vi "KV_CurHead_ReadCur.vi"(10 "地址":u8=1 max=10 step=1, 11 "MyIndex":u8) -> (3 "Value":dbl)   [LabVIEW 2015]
uses:
  <vilib>/Instr/_visa.llb/VISA Configure Serial Port (Instr).vi
panel:
  out "字符串":string
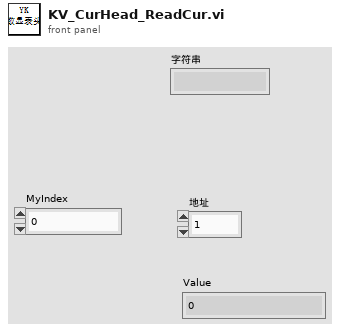
[diagram p1: front panel]
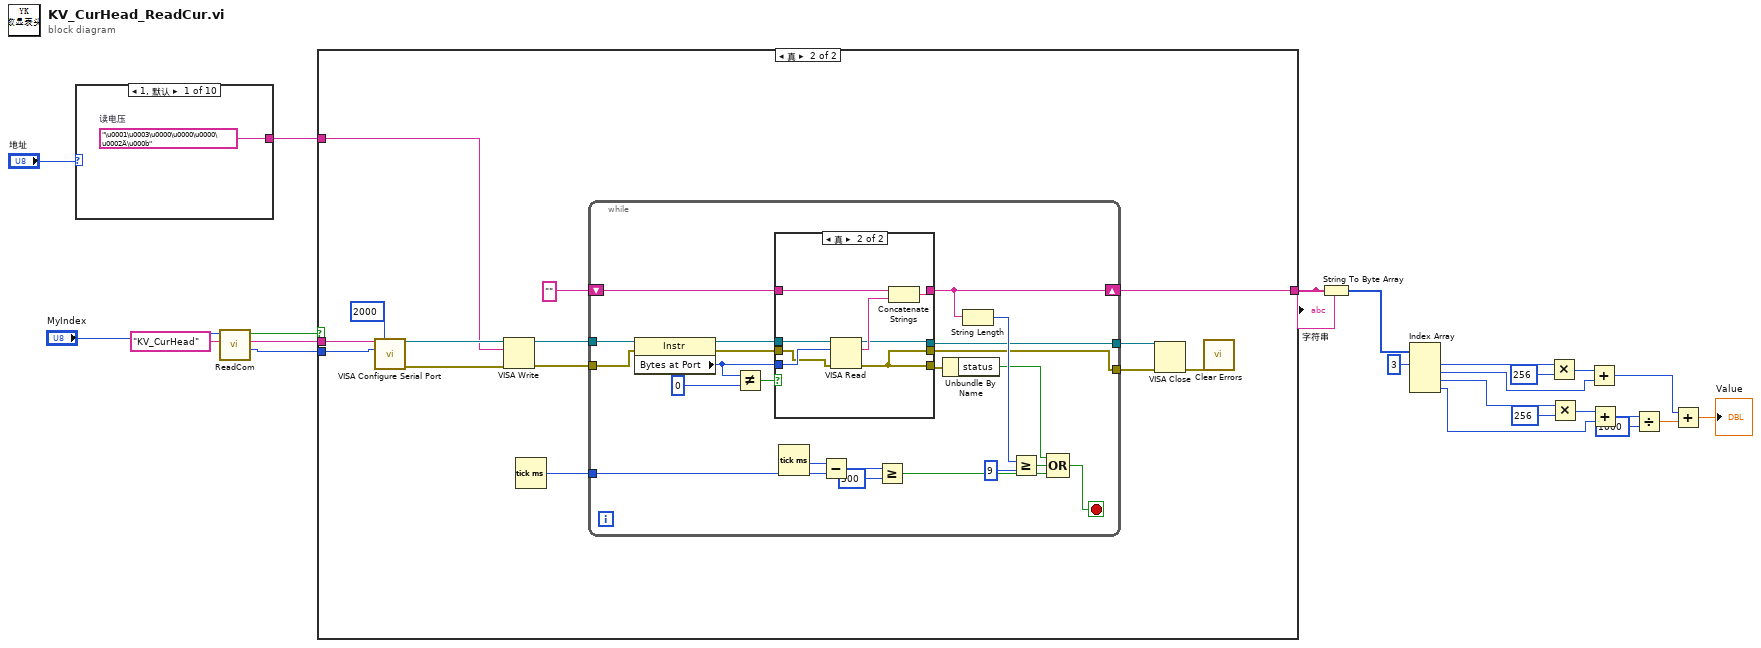
[diagram p0: block diagram]
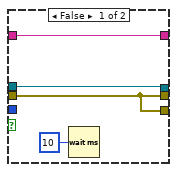
[diagram p3: hidden frame]
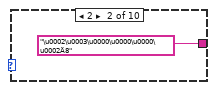
[diagram p4: hidden frame]
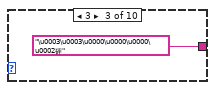
[diagram p5: hidden frame]
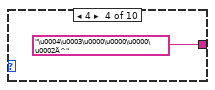
[diagram p6: hidden frame]
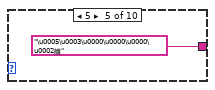
[diagram p7: hidden frame]
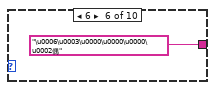
[diagram p8: hidden frame]
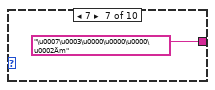
[diagram p9: hidden frame]
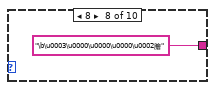
[diagram p10: hidden frame]
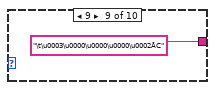
[diagram p11: hidden frame]
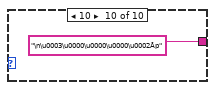
[diagram p12: hidden frame]
diagram:
  n1 = case shown="1, 默认" "地址" {
    tunnel: [w24 "\u0002\u0003\u0000\u0000\u0000\u0002Ä8" ("写入缓冲区") "\u0003\u0003\u0000\u0000\u0000\u0002砰" ("写入缓冲区") "\u0004\u0003\u0000\u0000\u0000\u0002Ä^" ("写入缓冲区") "\u0005\u0003\u0000\u0000\u0000\u0002艔" ("写入缓冲区") "\u0006\u0003\u0000\u0000\u0000\u0002偶" ("写入缓冲区") "\u0007\u0003\u0000\u0000\u0000\u0002Äm" ("写入缓冲区") "\b\u0003\u0000\u0000\u0000\u0002膾" ("写入缓冲区") "\t\u0003\u0000\u0000\u0000\u0002ÅC" ("写入缓冲区") "\n\u0003\u0000\u0000\u0000\u0002Åp" ("写入缓冲区")] -> w23
    frame 1, Default {
      w24 = "\u0001\u0003\u0000\u0000\u0000\u0002Ä\u000b"  # 读电压
    }
    frame 2 {
    }
    frame 3 {
    }
    frame 4 {
    }
    frame 5 {
    }
    frame 6 {
    }
    frame 7 {
    }
    frame 8 {
    }
    frame 9 {
    }
    frame 10 {
    }
  }
  n2 = call "ReadCom.vi"("仪器名称"="KV_CurHead", "MyIndex"="MyIndex") -> ("Baudrate"=w1:i32, "COM"=w3:string, "OK?"=w2:bool)  [unwired: 7 in]
  n3 = case shown="真" w2 {
    tunnel: w23 -> [_ w45]
    tunnel: [_ w40] -> w6
    tunnel: w3 -> [_ w38]
    tunnel: w1 -> [_ w34]
    frame False {
    }
    frame True {
      n4 = call-poly "VISA Configure Serial Port"("VISA resource name"=w38, "timeout (10sec)"=u32 2000, "baud rate (9600)"=w34) -> ("VISA resource name out"=w47:refnum<visa-resource-name>, "error out"=w46:errorcluster)  [unwired: 11 in]
      n5 = VISA Write(VISA resource name=w47, write buffer=w45, error in (no error)=w46) -> (VISA resource name out=w43:refnum<visa-resource-name>, error out=w44:errorcluster)  [unwired: 1 out]
      n6 = Tick Count (ms)() -> (millisecond timer value=w41:u32)
      n7 = while {
        tunnel: w44 -> [w48]
        tunnel: w43 -> [w69]
        shift-right: [w62] -> w40
        shift-left: "" -> [w63]
        tunnel: w41 -> [w54]
        tunnel: [w50] -> w37
        tunnel: [w49] -> w36
        stop <- w58 stop-if-true
        n8 = property class="Instr"(reference=w69, error in=w48) -> (reference out=w66:refnum<visa-resource-name>, error out=w64:errorcluster, "Bytes at Port"=w65:u32)
        n9 = Not Equal?(x=w65, y=u32 0) -> (x != y?=w67:bool)
        n10 = case shown="真" w67 {
          tunnel: w66 -> [w71 w81]
          tunnel: w65 -> [_ w80]
          tunnel: w64 -> [w70 w79]
          tunnel: w63 -> [w72 w78]
          tunnel: [w72 w76] -> w62
          tunnel: [w70 w74] -> w57
          tunnel: [w71 w75] -> w50
          tunnel: [w70 w74] -> w49
          frame False {
            n11 = Wait (ms)(milliseconds to wait=u32 10 ("等待时间（毫秒）")) -> ()  [unwired: 1 out]
          }
          frame True {
            n12 = VISA Read(VISA resource name=w81, byte count=w80, error in (no error)=w79) -> (VISA resource name out=w75:refnum<visa-resource-name>, read buffer=w77:string, error out=w74:errorcluster)  [unwired: 1 out]
            n13 = Concatenate Strings(w78, w77) -> (w76:string)
          }
        }
        n14 = Tick Count (ms)() -> (millisecond timer value=w55:u32)
        n15 = Subtract(x=w55, y=w54) -> (x-y=w53:u32)
        n16 = Greater Or Equal?(x=w53, y=u32 500) -> (x >= y?=w51:bool)
        n17 = Unbundle By Name(w57) -> ("status"=w56:bool)
        n18 = String Length(string=w62) -> (length=w61:i32)
        n19 = Greater Or Equal?(x=w61, y=9) -> (x >= y?=w60:bool)
        n20 = Compound Arithmetic op=OR ("复合运算")(w56, w60, w51) -> (w58:bool)
      }
      n21 = VISA Close(VISA resource name=w37, error in (no error)=w36) -> (error out=w35:errorcluster)
      n22 = call <vilib>:"Clear Errors.vi"("error in (no error)"=w35) -> ()  [unwired: 5 in, 2 out]
    }
  }
  "字符串" <- w6
  n23 = String To Byte Array(string=w6) -> (unsigned byte array=w8:u8[])
  n24 = Index Array(array=w8, index #1=3 ("索引")) -> (element #1=w21:u8, element #2=w18:u8, element #3=w15:u8, element #4=w14:u8)  [unwired: 3 in]
  n25 = Multiply(x=w21, y=i16 256) -> (x*y=w19:i16)
  n26 = Multiply(x=w15, y=i16 256) -> (x*y=w17:i16)
  n27 = Add(x=w19, y=w18) -> (x+y=w10:i16)
  n28 = Add(x=w17, y=w14) -> (x+y=w13:i16)
  n29 = Divide(x=w13, y=i16 1000) -> (x/y=w11:dbl)
  n30 = Add(x=w10, y=w11) -> (x+y=→"Value":dbl)
